vi "Connect.vi"(8 "error in (no error)":errorcluster, 11 "NI-DAQ in":refnum<class "NI-DAQ.lvclass">) -> (0 "error out":errorcluster, 3 "NI-DAQ out":refnum<class "NI-DAQ.lvclass">)   [LabVIEW 2021, in "NI-DAQ.lvclass"]
uses:
  NI-DAQ.lvclass
  NI-DAQ.lvclass/NI-DAQ.ctl
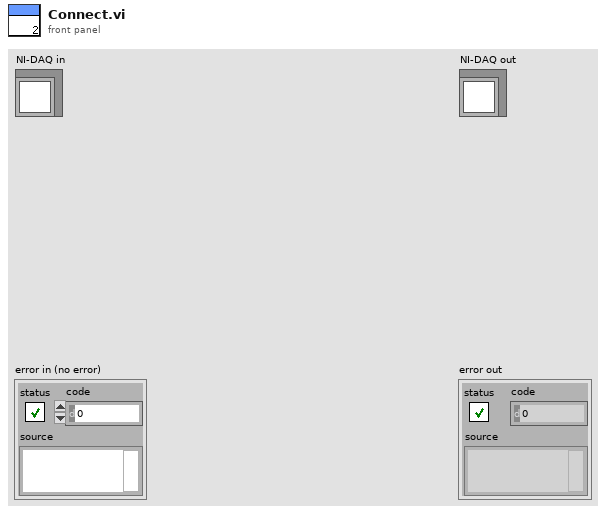
[diagram p1: front panel]
types:
  T1 = typedef "I-O.lvclass/Pin Map.ctl" = cluster{"Region Valves":i32[], "Extra Valves":dbl[][][], "Tool Primary Valve":i32, "Tool Secondary Valve":i32, "Region Sensors":i32[], "Extra Sensors":dbl[][][], "Tool Primary Sensor":dbl, "Tool Secondary Sensor":dbl, "Compression Sensor":dbl, "5V":i32, "Dispenser Sensor":dbl, "Light Curtain":i32}
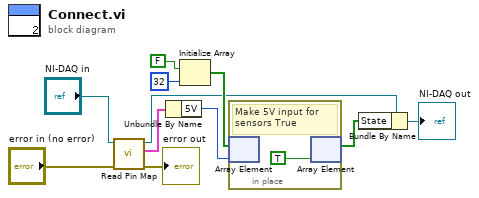
[diagram p0: block diagram]
diagram:
  n1 = call-dynamic "Read Pin Map.vi"("error in (no error)"="error in (no error)", "NI-DAQ in"="NI-DAQ in") -> ("error out"=→"error out":errorcluster, "Pin Map"=w4:T1, "NI-DAQ out"=w5:refnum<class "NI-DAQ.lvclass">)  [unwired: 7 in]
  n2 = Unbundle By Name(w4) -> ("5V"=w3:i32)
  n3 = Initialize Array(FALSE, 32 ("dimension size")) -> (w8:bool[])
  n4 = in-place {
    # "Make 5V input for sensors True"
    n5 = in-place-array #1(w8, w3) -> ()  [unwired: 1 out]
    n6 = in-place-array #1(TRUE) -> (w7:bool[])  [unwired: 1 out]
  }
  n7 = Bundle By Name(cluster=w5, "State"=w7) -> (→"NI-DAQ out":refnum<class "NI-DAQ.lvclass">)
